vi "Apply Theme To Splitter.vi"(7 "Override Root With (Empty)":string, 8 "Error In":errorcluster, 9 "Window Element":T1, 10 "Splitter Ref":refnum<vi>, 11 "ini Theme in":refnum<class "ini Theme.lvclass">) -> (0 "Error Out":errorcluster, 3 "ini Theme out":refnum<class "ini Theme.lvclass">)   [LabVIEW 2021, in "Appearance Actor.lvlib" / "ini Theme.lvclass"]
doc: "Apply theme to a <B>Splitter</B>. <B>Window Element</B> enum tells where it is on the window. <B>Override Root With</B> allows to override styling used for main window components."
uses:
  ini Theme.lvclass
  Generic Theme/API/Typedefs/Window Element--enum.ctl
  Generic Theme/API/Typedefs/Theme Control Property--enum.ctl
  ini Theme.lvclass/ini Theme.ctl
  7358f7a9-d3d2-4159-abff-5a45054637ef.vi
  3f727254-8c51-4e50-8872-a6056392d35e.vi
  7358f7a9-d3d2-4159-abff-5a45054637ef.vi/e124eda1-1651-4d76-919f-d33a8200b27b.vi
  7358f7a9-d3d2-4159-abff-5a45054637ef.vi/2055fcb7-c480-499a-9c31-028cc01b484e.vi
  3f727254-8c51-4e50-8872-a6056392d35e.vi/e124eda1-1651-4d76-919f-d33a8200b27b.vi
  3f727254-8c51-4e50-8872-a6056392d35e.vi/2055fcb7-c480-499a-9c31-028cc01b484e.vi
  Generic Theme/API/Utilities/Theme Entry Enum To String.vi
  Generic Theme/API/Constants/Default Entry Value--String.vi
  <vilib>/Utility/config.llb/Read Key.vi
  <vilib>/Utility/config.llb/Read Key (String).vi
  <vilib>/Utility/config.llb/NI_LVConfig.lvlib
  Generic Theme/Generic Theme.lvclass
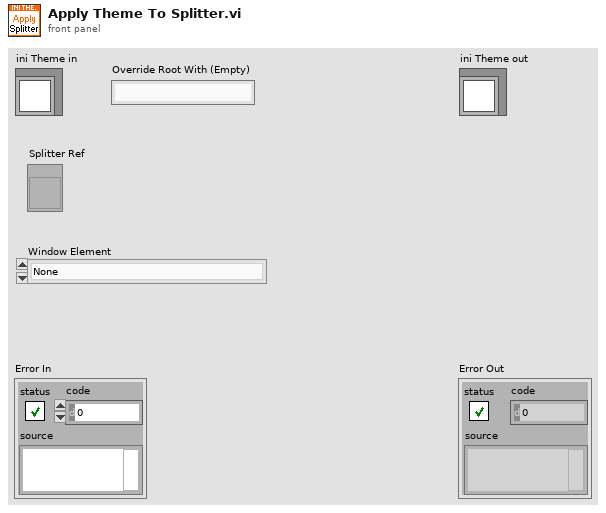
[diagram p1: front panel]
types:
  T1 = typedef "Appearance Actor.lvlib/Generic Theme.lvclass/Window Element--enum.ctl" = enum16{"None", "TB", "SM", "BP", "SB"}
  T2 = typedef "Appearance Actor.lvlib/Generic Theme.lvclass/Theme Control Property--enum.ctl" = enum16{"None", "Button.FalseFillColor", "Button.FalseOutlineColor", "Button.FalseToTrueFillColor", "Button.FalseToTrueOutlineColor", "Button.HoverFalseFillColor", "Button.HoverFalseOutlineColor", "Button.HoverTrueFillColor", "Button.HoverTrueOutlineColor", "Button.TrueFillColor", "Button.TrueOutlineColor", "Button.TrueToFalseFillColor", "Button.TrueToFalseOutlineColor", "CloseButton.FalseFillColor", "CloseButton.FalseOutlineColor", "CloseButton.FalseToTrueFillColor", "CloseButton.FalseToTrueOutlineColor", "CloseButton.HoverFalseFillColor", "CloseButton.HoverFalseOutlineColor", "CloseButton.HoverTrueFillColor", "CloseButton.HoverTrueOutlineColor", "CloseButton.TrueFillColor", "CloseButton.TrueOutlineColor", "CloseButton.TrueToFalseFillColor", "CloseButton.TrueToFalseOutlineColor", "Pane.Color", "Splitter.FillColor", "Splitter.OutlineColor", "Splitter.Size", "Title.Font.Color", "Title.Font.Family", "Title.Font.Size", "Title.Font.Style"}
  T3 = typedef "NI_LVConfig.lvlib/Config Data RefNum.ctl" = refnum<k1>
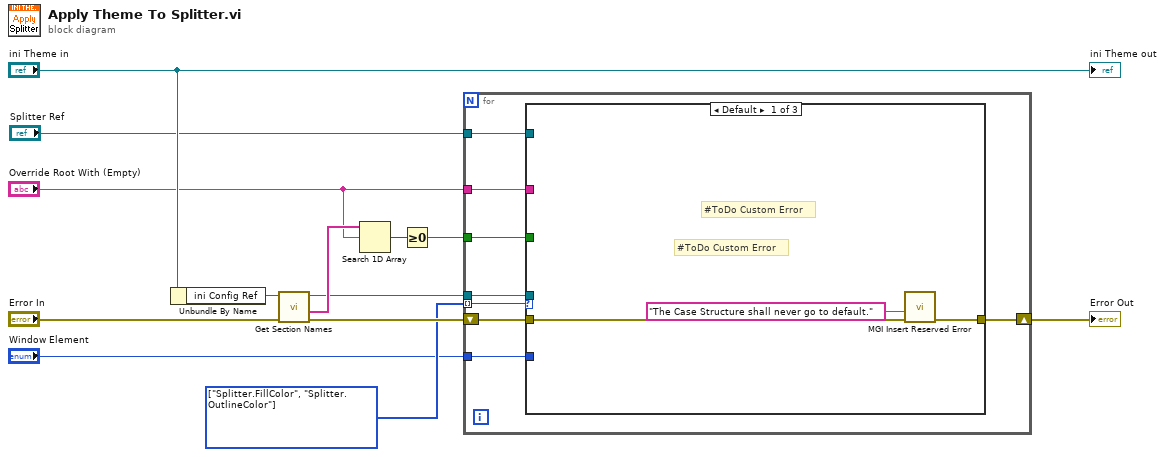
[diagram p0: block diagram]
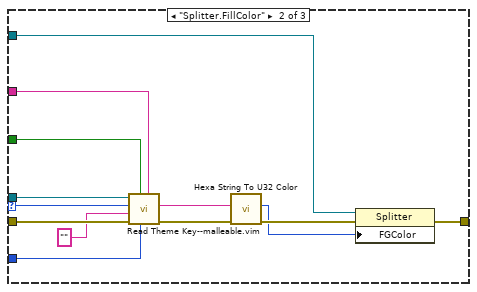
[diagram p2: hidden frame]
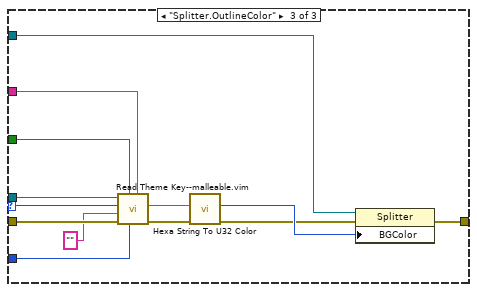
[diagram p3: hidden frame]
diagram:
  w3 = T2[] [enum."Splitter.FillColor", enum."Splitter.OutlineColor"] items=["None", "Button.FalseFillColor", "Button.FalseOutlineColor", "Button.FalseToTrueFillColor", "Button.FalseToTrueOutlineColor", "Button.HoverFalseFillColor", "Button.HoverFalseOutlineColor", "Button.HoverTrueFillColor", "Button.HoverTrueOutlineColor", "Button.TrueFillColor", "Button.TrueOutlineColor", "Button.TrueToFalseFillColor", "Button.TrueToFalseOutlineColor", "CloseButton.FalseFillColor", "CloseButton.FalseOutlineColor", "CloseButton.FalseToTrueFillColor", "CloseButton.FalseToTrueOutlineColor", "CloseButton.HoverFalseFillColor", "CloseButton.HoverFalseOutlineColor", "CloseButton.HoverTrueFillColor", "CloseButton.HoverTrueOutlineColor", "CloseButton.TrueFillColor", "CloseButton.TrueOutlineColor", "CloseButton.TrueToFalseFillColor", "CloseButton.TrueToFalseOutlineColor", "Pane.Color", "Splitter.FillColor", "Splitter.OutlineColor", "Splitter.Size", "Title.Font.Color", "Title.Font.Family", "Title.Font.Size", "Title.Font.Style"] ("Array")
  n1 = Unbundle By Name("ini Theme in") -> ("ini Config Ref"=w13:T3)
  n2 = call <vilib>:"Get Section Names.vi"("error in (no error)"="Error In", "refnum"=w13) -> ("error out"=w10:errorcluster, "section names"=w12:string[], "refnum out"=w4:T3)  [unwired: 7 in]
  n3 = Search 1D Array(1D array=w12, element="Override Root With (Empty)") -> (index of element=w11:i32)  [unwired: 1 in]
  n4 = Greater Or Equal To 0?(x=w11) -> (x >= 0?=w5:bool)
  n5 = for {
    shift-right: [w16] -> w8
    shift-left: w10 -> [w21]
    tunnel: "Override Root With (Empty)" -> [w20]
    tunnel: w5 -> [w19]
    tunnel: w4 -> [w18]
    tunnel: w3 -> [w17] mode=indexing
    tunnel: "Splitter Ref" -> [w15]
    tunnel: "Window Element" -> [w14]
    n6 = case shown="Default" w17 {
      selector: w17 -> [_ w33 w44]
      tunnel: w21 -> [w23 w34 w46]
      tunnel: w20 -> [_ w29 w38]
      tunnel: w19 -> [_ w30 w39]
      tunnel: w18 -> [_ w31 w45]
      tunnel: [w22 w36 w48] -> w16
      tunnel: w15 -> [_ w35 w47]
      tunnel: w14 -> [_ w25 w37]
      frame Default {
        # "#ToDo Custom Error"
        # "#ToDo Custom Error"
        n7 = call <userlib>:"MGI Insert Reserved Error.vi"("Error In"=w23, "Error Description"="The Case Structure shall never go to default.") -> ("Error Out"=w22:errorcluster)  [unwired: 9 in]
      }
      frame "Splitter.FillColor" {
        n8 = call "Read Theme Key--malleable.vim"("Section for Override (Empty)"=w29, "Window Element"=w25, "Can Be Overriden (F)"=w30, "Error In"=w34, "Data Type"="", "Theme Control Property"=w33, "ini Ref In"=w31) -> ("Error Out"=w28:errorcluster, "Value"=w26:string)  [unwired: 2 in, 1 out]
        n9 = call "Hexa String To U32 Color.vi"("8 Char Hexa String"=w26) -> ("U32 Color"=w27:u32)  [unwired: 10 in]
        n10 = property class="Splitter"(reference=w35, error in=w28, "FGColor"=w27) -> (error out=w36:errorcluster)  [unwired: 1 out]
      }
      frame "Splitter.OutlineColor" {
        n11 = call "Read Theme Key--malleable.vim"("Section for Override (Empty)"=w38, "Window Element"=w37, "Can Be Overriden (F)"=w39, "Error In"=w46, "Data Type"="", "Theme Control Property"=w44, "ini Ref In"=w45) -> ("Error Out"=w40:errorcluster, "Value"=w42:string)  [unwired: 2 in, 1 out]
        n12 = call "Hexa String To U32 Color.vi"("8 Char Hexa String"=w42) -> ("U32 Color"=w41:u32)  [unwired: 10 in]
        n13 = property class="Splitter"(reference=w47, error in=w40, "BGColor"=w41) -> (error out=w48:errorcluster)  [unwired: 1 out]
      }
    }
  }
  "Error Out" <- w8
  "ini Theme out" <- "ini Theme in"
